vi "Test Bench Constants Linux x64.vi"() -> (1 "Deployment Hooks class":refnum<class "Custom Device Deployment Hooks.lvclass">, 3 "Custom Device class":refnum<class "Custom Device.lvclass">)   [LabVIEW 2026]
uses:
  <userlib>/Custom Device Interfaces_v1.lvlibp/CustomDevice/Custom Device.lvclass
  <userlib>/Custom Device Interfaces_v1.lvlibp/CustomDeviceDeploymentHooks/Custom Device Deployment Hooks.lvclass
  Engine/SystemMonitor Engine.lvclass
  C:/SysMon1/SystemMonitor Custom Device/SystemMonitor/Engine/SystemMonitor Engine.lvclass
  C:/Program Files/NI/LVAddons/nivscustomdeviceexpress/1/Targets/NI/RT/Linux/PXI/user.lib/Custom Device Interfaces_v1.lvlibp/CustomDevice/Custom Device.lvclass
  Deployment Hooks/SystemMonitor Deployment Hooks.lvclass
  C:/SysMon1/SystemMonitor Custom Device/SystemMonitor/Deployment Hooks/SystemMonitor Deployment Hooks.lvclass
  C:/Program Files/NI/LVAddons/nivscustomdeviceexpress/1/Targets/NI/RT/Linux/PXI/user.lib/Custom Device Interfaces_v1.lvlibp/CustomDeviceDeploymentHooks/Custom Device Deployment Hooks.lvclass
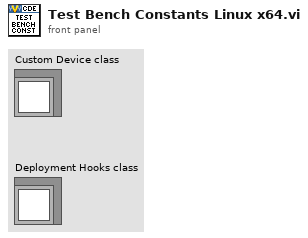
[diagram p1: front panel]
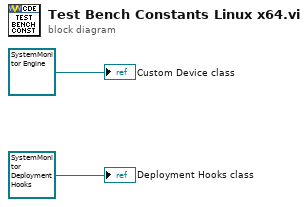
[diagram p0: block diagram]
diagram:
  "Custom Device class" <- refnum<class "SystemMonitor Engine.lvclass"> refnum ("SystemMonitor Engine.lvlib:SystemMonitor Engine.lvclass")
  "Deployment Hooks class" <- refnum<class "SystemMonitor Deployment Hooks.lvclass"> refnum ("SystemMonitor Deployment Hooks.lvlib:SystemMonitor Deployment Hooks.lvclass")
